vi "XY Graph Shift Plot.vi"(6 "Plot Shift Parameters":T1 caption="IRF Analysis Parameters", 7 "Reference Decay":cluster{"t Array":dbl[], "I Array":dbl[]}, 8 "error in (no error)":errorcluster, 9 "Replace Plot (T)?":bool=TRUE, 11 "Selected Plot Info":T3={"Multiplot XY Graph"=refnum, "Mouse Coordinates"={"Horizontal"=0, "Vertical"=0}, "Plot Index"=-1}) -> (0 "Error Out":errorcluster, 1 "Shift Decay Message":string, 3 "Shifted Plot":cluster{"t Array":dbl[], "IRF Array":dbl[]})   [LabVIEW 2021, in "XY Graph Add-Ons.lvlib"]
uses:
  XY Graph Add-Ons.lvlib
  XY Graph Selected Plot Info.ctl
  XY Graph Refnum.ctl
  <vilib>/Utility/miscctls.llb/LVPoint32TypeDef.ctl
  XY Graph Plot Shift Parameters.ctl
  XY Graph Plot Shift Method.ctl
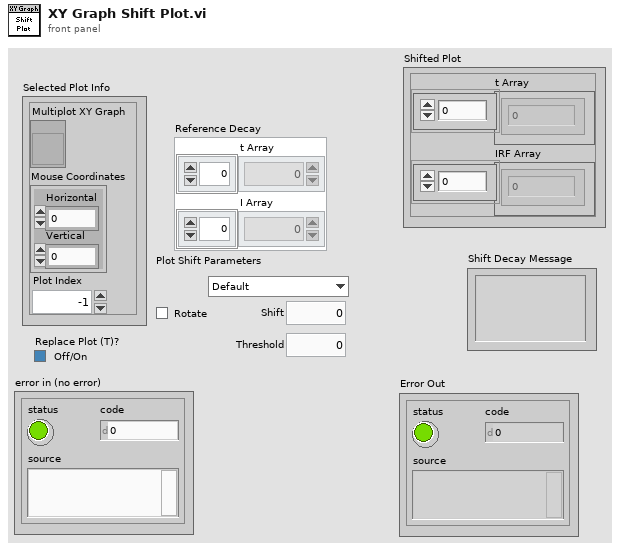
[diagram p1: front panel]
types:
  T1 = typedef "XY Graph Add-Ons.lvlib/XY Graph Plot Shift Parameters.ctl" = cluster{"Type":T2, "Shift":dbl[unit], "Threshold":dbl, "Rotate":bool}
  T2 = typedef "XY Graph Add-Ons.lvlib/XY Graph Plot Shift Method.ctl" = enum16{"Default", "CFD", "Threshold", "Cross-Correlation"}
  T3 = typedef "XY Graph Add-Ons.lvlib/XY Graph Selected Plot Info.ctl" = cluster{"Multiplot XY Graph":T4, "Mouse Coordinates":T5, "Plot Index":i32}
  T4 = typedef "XY Graph Add-Ons.lvlib/XY Graph Refnum.ctl" = refnum<vi>
  T5 = typedef "LVPoint32TypeDef.ctl" = cluster{"Horizontal":i32, "Vertical":i32}
  T6 = cluster{"t Axis":dbl[], "ROI Intensity Array in":dbl[]}
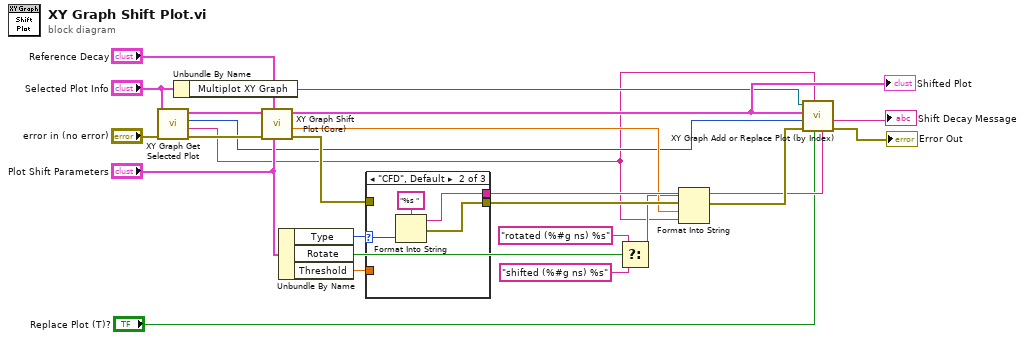
[diagram p0: block diagram]
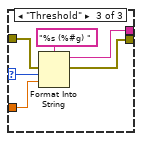
[diagram p3: hidden frame]
diagram:
  n1 = call "XY Graph Get Selected Plot.vi"("error in (no error)"="error in (no error)", "Selected Plot Info"="Selected Plot Info") -> ("error out"=w10:errorcluster, "Plot Name"=w3:string, "Plot Index"=w8:i32, "Plot"=w9:cluster{"X Array":dbl[], "Y Array":dbl[]})  [unwired: 4 in, 2 out]
  n2 = Unbundle By Name("Selected Plot Info") -> ("Multiplot XY Graph"=w6:T4)
  n3 = call "XY Graph Shift Plot (Core).vi"("Plot Shift Parameters"="Plot Shift Parameters", "Time-Gated Reference Decay"="Reference Decay", "error in (no error)"=w10, "Decay in"=w9) -> ("error out"=w17:errorcluster, "Shift (ns)"=w16:dbl, "Decay out"=w13:T6)  [unwired: 5 in]
  "Shifted Plot" <- w13
  n4 = Unbundle By Name("Plot Shift Parameters") -> ("Type"=w21:T2, "Rotate"=w22:bool, "Threshold"=w18:dbl)
  n5 = case shown="\"CFD\", Default" w21 {
    selector: w21 -> [_ w30 w36]
    tunnel: [_ w27 w33] -> w20
    tunnel: [w26 w28 w34] -> w19
    tunnel: w18 -> [_ _ w32]
    tunnel: w17 -> [w26 _ w31]
    frame "Default" {
    }
    frame "CFD", Default {
      n6 = Format Into String(format string="%s ", w30) -> (resulting string=w27:string, error out=w28:errorcluster)  [unwired: 2 in]
    }
    frame "Threshold" {
      n7 = Format Into String(format string="%s (%#g) ", error in=w31, w36, w32) -> (resulting string=w33:string, error out=w34:errorcluster)  [unwired: 1 in]
    }
  }
  n8 = Select(t="rotated (%#g ns) %s" ("string"), s=w22, f="shifted (%#g ns) %s" ("string")) -> (s? t:f=w15:string)
  n9 = Format Into String(format string=w15, initial string=w20, error in=w19, w16, w3) -> (resulting string=w2:string, error out=w12:errorcluster)
  n10 = call "XY Graph Add or Replace Plot (by Index).vi"("New Plot Name"=w2, "Replace Plot (T)?"="Replace Plot (T)?", "Original Plot Name"=w3, "error in (no error)"=w12, "Plot Index"=w8, "Plot in"=w13, "XYGraph in"=w6) -> ("error out"=→"Error Out":errorcluster, "Message"=→"Shift Decay Message":string)  [unwired: 3 in]
